vi "SS2 Live_Get Single Image Set.vi"(8 "error in (no error)":errorcluster, 11 "SS2 Live Internal Variables":T1={"okCFrontPanelDevices Refnum"=refnum, "Device Refnum"=refnum, "Display Image"=refnum, "# Live Images"=0, "relative s"=0.0, "# Image Sets"=0, "Message"="", "Current Image Set"=0, "# Datasets"=0, "Current Dataset"=0, "Live Mode"=FALSE, "Recording Mode"=FALSE, "Record Button"=refnum, "Live Button"=refnum, "SS2 Live Gate Data Q Name"="SS2 Live Gate Data Q", "Discard First Image"=FALSE, "Image Information"={"Save ROI Only"=FALSE, "Left"=0, "Top"=0, "Right"=0, "Bottom"=0, "Use Current ROI"=FALSE}, "Image Binning Options"={"Use Image Binning"=FALSE, "X Bin"=1, "Y Bin"=1}, "FPGA Serial Number"="", "PCB Version"=enum."PCB 1"} {"Image Binning Options"."Y Bin" min=1; "Image Binning Options"."X Bin" min=1}) -> (0 "error out":errorcluster, 3 "SS2 Live Internal Variables out":T1={"okCFrontPanelDevices Refnum"=refnum, "Device Refnum"=refnum, "Display Image"=refnum, "# Live Images"=0, "relative s"=0.0, "# Image Sets"=0, "Message"="", "Current Image Set"=0, "# Datasets"=0, "Current Dataset"=0, "Live Mode"=FALSE, "Recording Mode"=FALSE, "Record Button"=refnum, "Live Button"=refnum, "SS2 Live Gate Data Q Name"="SS2 Live Gate Data Q", "Discard First Image"=FALSE, "Image Information"={"Save ROI Only"=FALSE, "Left"=0, "Top"=0, "Right"=0, "Bottom"=0, "Use Current ROI"=FALSE}, "Image Binning Options"={"Use Image Binning"=FALSE, "X Bin"=1, "Y Bin"=1}, "FPGA Serial Number"="", "PCB Version"=enum."PCB 1"} {"Image Binning Options"."Y Bin" min=1; "Image Binning Options"."X Bin" min=1})   [LabVIEW 2019]
uses:
  SS2 Live Internal Variables.ctl
  C:/UCLA Thinkpad Google Drive/LabVIEW 2019 SP1/builds/SS2 Live Distribution/Opal Kelly/C# Wrapper/libFrontPanel-csharp.dll
  Opal Kelly/C# Wrapper/libFrontPanel-csharp.dll
  <vilib>/vision/Image Controls.llb/IMAQ Image.ctl
  SS2 Live_Image ROI Information.ctl
  Phasor/Image Binning Options.ctl
  SS2 DAQ PCB Version.ctl
  SS2 Live_Settings List.ctl
  Variant/Variant to Data/Variant to Data.lvlib
panel:
  out "init FPGA Error Out":errorcluster
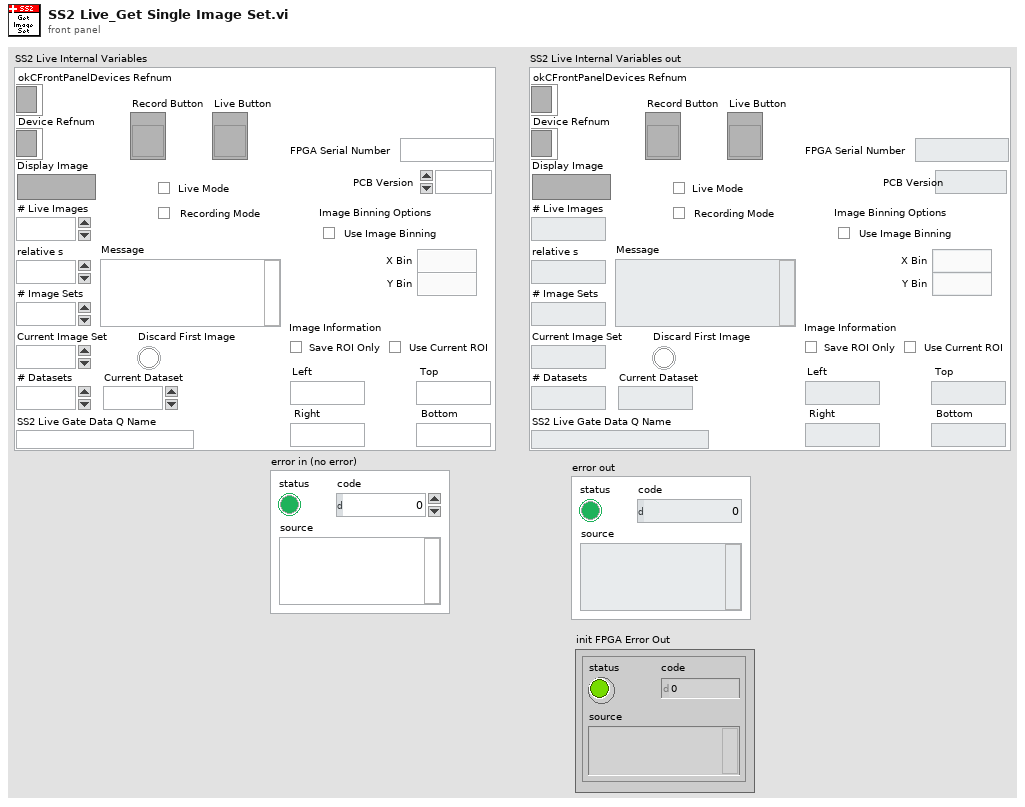
[diagram p1: front panel]
types:
  T1 = typedef "SS2 Live Internal Variables.ctl" = cluster{"okCFrontPanelDevices Refnum":refnum<k24>, "Device Refnum":refnum<k24>, "Display Image":T2, "# Live Images":i32, "relative s":dbl, "# Image Sets":i32, "Message":string, "Current Image Set":i32, "# Datasets":i32, "Current Dataset":i32, "Live Mode":bool, "Recording Mode":bool, "Record Button":refnum<vi>, "Live Button":refnum<vi>, "SS2 Live Gate Data Q Name":string, "Discard First Image":bool, "Image Information":T3, "Image Binning Options":T4, "FPGA Serial Number":string, "PCB Version":T5}
  T2 = typedef "IMAQ Image.ctl" = refnum<image>
  T3 = typedef "SS2 Live_Image ROI Information.ctl" = cluster{"Save ROI Only":bool, "Left":u16, "Top":u16, "Right":u16, "Bottom":u16, "Use Current ROI":bool}
  T4 = typedef "Image Binning Options.ctl" = cluster{"Use Image Binning":bool, "X Bin":i32, "Y Bin":i32}
  T5 = typedef "SS2 DAQ PCB Version.ctl" = enum16{"unknown", "PCB 1", "PCB 2"}
  T6 = typedef "SS2 Live_Settings List.ctl" = enum16{"FPGA:Bitfile Path", "FPGA:Bitfile Version", "FPGA:Auto Reset FPGA", "Acquisition Parameters:SS2 DAQ Parameters", "Acquisition Parameters:Gate Configuration Array", "Acquisition Parameters:Buffer Size (# Gates)", "File Information:File Information", "File Information:# Datasets in Series", "File Information:Scrambled File Flag", "File Information:Delay between Datasets", "Image Parameters:Image ROI Information", "Image Parameters:Image Binning Options", "UI Settings:Histogram Bins Number"}
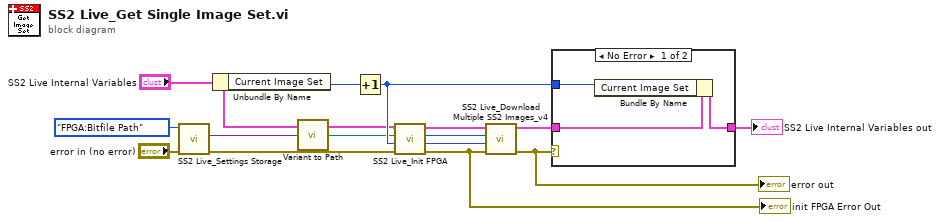
[diagram p0: block diagram]
diagram:
  n1 = call "SS2 Live_Settings Storage.vi"("Error In"="error in (no error)", "Settings List"=SS2_Live_Settings_List."FPGA:Bitfile Path") -> ("Error Out"=w12:errorcluster, "Variant Data out"=w14:variant)  [unwired: 8 in]
  n2 = Unbundle By Name("SS2 Live Internal Variables") -> ("Current Image Set"=w15:i32)
  n3 = call "Variant to Path.vi"("Variant"=w14) -> ("Path"=w9:path)  [unwired: 8 in]
  n4 = Increment(x=w15) -> (x+1=w10:i32)
  n5 = call "SS2 Live_Init FPGA.vi"("Error In"=w12, "Current Image Set"=w10, "FPGA bitfile Path"=w9, "SS2 Live Internal Variables in"="SS2 Live Internal Variables") -> ("Error Out"=w7:errorcluster, "# 8-bit Images per Set"=w1:u32, "Buffer Size (#8-bit Images)"=w2:u32, "SS2 Live Internal Variables out"=w4:T1)  [unwired: 4 in]
  "init FPGA Error Out" <- w7
  n6 = call "SS2 Live_Download Multiple SS2 Images_v4.vi"("Error In"=w7, "# 8-bit Images (1)"=w1, "Buffer Size (#8-bit Images)"=w2, "SS2 Live Internal Variables"=w4) -> ("Error Out"=w6:errorcluster, "SS2 Live Internal Variables"=w3:T1)  [unwired: 6 in]
  "error out" <- w6
  n7 = case shown="No Error" w6 {
    tunnel: w3 -> [w18 w19]
    tunnel: [w17 w19] -> w11
    tunnel: w10 -> [w16 _]
    frame No Error {
      n8 = Bundle By Name(cluster=w18, "Current Image Set"=w16) -> (w17:T1)
    }
    frame Error {
    }
  }
  "SS2 Live Internal Variables out" <- w11
